vi "PWM Calibration INI File.vi"(8 "error in (no error)":errorcluster, 9 "Driver":T1, 10 "Operation":T2, 11 "Calibration In":T3) -> (0 "error out":errorcluster, 2 "Calibration Out":T3)   [LabVIEW 2011]
uses:
  PWM Normalization State.ctl
  Calibration INI File Command.ctl
  Calibration INI File Driver.ctl
  <vilib>/Utility/config.llb/Read Key (String).vi
  <vilib>/Utility/config.llb/Write Key (String).vi
  <vilib>/Utility/config.llb/NI_LVConfig.lvlib
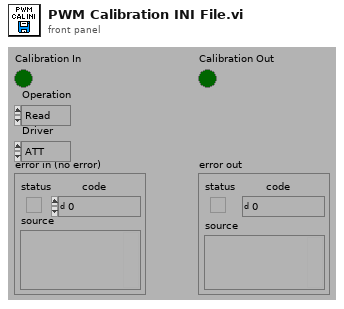
[diagram p1: front panel]
types:
  T1 = typedef "Calibration INI File Driver.ctl" = enum16{"ATT", "DMM", "IMP", "PFE", "PIM", "PWM", "SNA", "SWI", "VNA"}
  T2 = typedef "Calibration INI File Command.ctl" = enum16{"Read", "Write", "Clear"}
  T3 = typedef "PWM Normalization State.ctl" = bool
  T4 = typedef "NI_LVConfig.lvlib/Config Data RefNum.ctl" = refnum<k1>
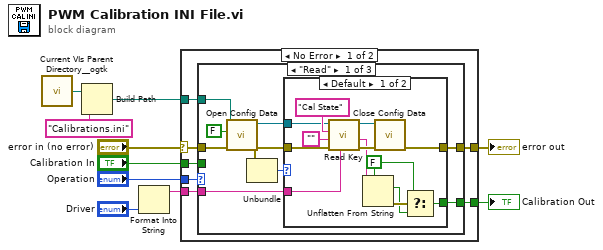
[diagram p0: block diagram]
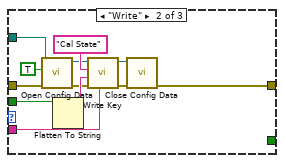
[diagram p3: hidden frame]
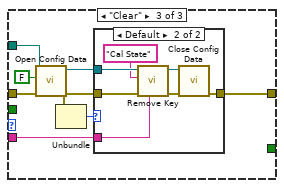
[diagram p4: hidden frame]
diagram:
  n1 = call "Current VIs Parent Directory__ogtk.vi"() -> ("Parent Directory (+ Relative)"=w3:path)  [unwired: 5 in]
  n2 = Build Path(base path=w3, name or relative path="Calibrations.ini") -> (appended path=w9:path)
  n3 = Format Into String("Driver") -> (resulting string=w2:string)  [unwired: 3 in, 1 out]
  n4 = case shown="No Error" "error in (no error)" {
    selector: "error in (no error)" -> [w12 w67]
    tunnel: w9 -> [w17 _]
    tunnel: [w16 w67] -> w8
    tunnel: [w15 _] -> w7
    tunnel: "Operation" -> [w14 _]
    tunnel: "Calibration In" -> [w13 _]
    tunnel: w2 -> [w11 _]
    frame No Error {
      n5 = case shown="\"Read\"" w14 {
        tunnel: w17 -> [w23 w43 w55]
        tunnel: w12 -> [w22 w44 w54]
        tunnel: [w26 w42 w53] -> w16
        tunnel: [w25 _ _] -> w15
        tunnel: w13 -> [_ w41 _]
        tunnel: w11 -> [w18 w40 w52]
        frame "Read" {
          n6 = call <vilib>:"Open Config Data.vi"("error in (no error)"=w22, "create file if necessary (T)"=FALSE ("create file if necessary? (T)"), "configuration file path"=w23) -> ("error out"=w21:errorcluster, "refnum"=w24:T4)  [unwired: 6 in, 1 out]
          n7 = Unbundle(w21) -> ("code"=w20:i32)  [unwired: 2 out]
          n8 = case shown="Default" w20 {
            tunnel: w21 -> [w33 _]
            tunnel: [w39 _] -> w26
            tunnel: w24 -> [w32 _]
            tunnel: [w27 _] -> w25
            tunnel: w18 -> [w31 _]
            frame Default {
              w28 = T3 FALSE ("Calibration")
              n9 = call-poly <vilib>:"Read Key.vi"("section"=w31, "error in (no error)"=w33, "default value"="", "key"="Cal State" ("format string"), "refnum"=w32) -> ("error out"=w37:errorcluster, "value"=w35:string, "refnum out"=w38:T4)  [unwired: 1 in, 3 out]
              n10 = Unflatten From String(type=w28, binary string=w35) -> (value=w29:T3, error out=w30:errorcluster)  [unwired: 1 in, 3 out]
              n11 = call <vilib>:"Close Config Data.vi"("error in (no error)"=w37, "refnum"=w38) -> ("error out"=w39:errorcluster)  [unwired: 1 in, 8 out]
              n12 = Select(t=w28, s=w30, f=w29) -> (s? t:f=w27:T3)
            }
            frame 7 {
            }
          }
        }
        frame "Write" {
          n13 = call <vilib>:"Open Config Data.vi"("error in (no error)"=w44, "create file if necessary (T)"=TRUE ("create file if necessary? (T)"), "configuration file path"=w43) -> ("error out"=w46:errorcluster, "refnum"=w47:T4)  [unwired: 6 in, 1 out]
          n14 = Flatten To String(anything=w41) -> (data string=w50:string)  [unwired: 1 in, 4 out]
          n15 = call-poly <vilib>:"Write Key.vi"("section"=w40, "error in (no error)"=w46, "value"=w50, "key"="Cal State" ("format string"), "refnum"=w47) -> ("error out"=w48:errorcluster, "refnum out"=w49:T4)  [unwired: 1 in, 4 out]
          n16 = call <vilib>:"Close Config Data.vi"("error in (no error)"=w48, "refnum"=w49) -> ("error out"=w42:errorcluster)  [unwired: 1 in, 8 out]
        }
        frame "Clear" {
          n17 = call <vilib>:"Open Config Data.vi"("error in (no error)"=w54, "create file if necessary (T)"=FALSE ("create file if necessary? (T)"), "configuration file path"=w55) -> ("error out"=w57:errorcluster, "refnum"=w59:T4)  [unwired: 6 in, 1 out]
          n18 = Unbundle(w57) -> ("code"=w56:i32)  [unwired: 2 out]
          n19 = case shown="Default" w56 {
            tunnel: w57 -> [_ w66]
            tunnel: w59 -> [_ w65]
            tunnel: [_ w64] -> w53
            tunnel: w52 -> [_ w60]
            frame 7 {
            }
            frame Default {
              n20 = call <vilib>:"Remove Key.vi"("section"=w60, "error in (no error)"=w66, "key"="Cal State" ("name or relative path"), "refnum"=w65) -> ("error out"=w62:errorcluster, "refnum out"=w61:T4)  [unwired: 6 out]
              n21 = call <vilib>:"Close Config Data.vi"("error in (no error)"=w62, "refnum"=w61) -> ("error out"=w64:errorcluster)  [unwired: 1 in, 8 out]
            }
          }
        }
      }
    }
    frame Error {
    }
  }
  "error out" <- w8
  "Calibration Out" <- w7
